vi "SYST_PRES.vi"(0 "VISA IN":refnum<visa-resource-name>, 5 "error in":errorcluster) -> (14 "VISA Out":refnum<visa-resource-name>, 19 "error out":errorcluster)   [LabVIEW 2018, in "PNA-X.lvlib"]
doc: "SYSTem:PRESet. The contents of the analyzer's non-volatile memory are not affected by this \ncommand. \n*SRE - Service Request Enable \nBefore reading a status register, bits must be enabled. This command enables bits in the service request \nregister. The current setting is saved in non-volatile memory. See Status Commands and Reading the \nAnalyzer's Status Registers. \n*SRE? - Service Request Enable Query \nReads the current state of the service request enable register. The register is cleared after reading it. The \nreturn value can be decoded using the table in Status Commands. See also Reading the Analyzer's \n1483\n\nStatus Registers. \n*STB? - Status Byte Query \nReads the value of the instrument status byte. The register is cleared only when the registers feeding it \nare cleared. See Status Commands and Reading the Analyzer's Status Registers. \n*TST? - Result of Self-test Query \nReturns the result of a query of the analyzer hardward status. An 0 indicates no failures found. Any \nother value indicates one or more of the following conditions exist. The value returned is the Weight \n(or sum of the Weights) of the existing conditions. For example: \nIf 4 is returned from *TST?, an Overpower condition exists. \nIf 6 is returned, both Unleveled and Overpower conditions exists. \nBit Weight Description Bit is set to 1 when the following conditions exist: \n0 1 Phase Unlock The source has lost phaselock. This could be caused by a \nreference channel open or a hardware failure. \n1 2 Unleveled The source power is unleveled. This could be a source is set \nfor more power than it can deliver at the tuned frequency. Or \nit could be caused by a hardware failure. \n2 4 Not used \n3 8 EE Write Failed An attempted write to the EEPROM has failed. This is \npossibly caused by a hardware failure. \n4 16 YIG Cal Failed The analyzer was unable to calibrate the YIG. Either the \nphaselock has been lost or there has been a hardware failure. \n5 32 Ramp Cal Failed The analyzer was unable to calibrate the analog ramp \ngenerator due to a possible hardware failure. \n6 64 Not used \n*WAI - Wait \nProhibits the instrument from executing any new commands until all pending overlapped commands \nhave been completed. See Understanding Command Synchronization \n1484\n\nAbout Triggering \nAbort Command \nABORt \n(Write-only) Stops all sweeps - then resume per current trigger settings. This command is the same as \nINITtiate:IMMediate (restart) except if a channel is performing a single sweep, ABORt will stop the \nsweep, but not initiate another sweep. \nLearn about Synchronizing the PNA and Controller \nExamples ABOR \nabort \nQuery Syntax Not applicable \nDefault Not applicable \n1485\n\nCalculate:Correction Commands \nControls error correction functions. \nClick on a blue keyword to view the command details. \nSee Also \nExample Programs \nNew Calibrating the PNA Using SCPI \nSynchronizing the PNA and Controller \nSCPI Command Tree \nCritical Note: CALCulate commands act on the selected measurement. You can select one \nmeasurement for each channel using Calc:Par:Select \nCALCulate<cnum>:CORRection:EDELay:MEDium <char> \n(Read-Write) Sets the media used when calculating the electrical delay. \nParameters \n<cnum> Any existing channel number. If unspecified, value is set to 1. \n<num> Choose from: COAX for coaxial medium, WAVEguide for waveguide \nmedium. \nExamples CALC:CORR:EDEL:MED COAX \ncalc3:corr:edelay:medium waveguide \nQuery Syntax CALCulate<cnum>:CORRection:EDELay:MEDium? \nReturn Type Character \nDefault COAX \n1486\n\nCALCulate<cnum>:CORRection:EDELay:TIME <num> \n(Read-Write) Sets the electrical delay for the selected measurement. \nSee Critical Note \nParameters \n<cnum> Channel number of the measurement. There must be a selected measurement \non that channel. If unspecified, <cnum> is set to 1. \n<num> Electrical delay in seconds. Choose any number between: \n-10.00 and 10.00 \nUse SENS:CORR:RVEL:COAX <num> to set Velocity factor. \nExamples CALC1:CORR:EDEL:TIME 1NS \ncalculate2:correction:time 0.5e-12 \nQuery Syntax CALCulate:CORRection:EDELay:TIME? \nReturn Type Numeric \nDefault 0 seconds \nCALCulate<cnum>:CORRection:EDELay:WGCutoff <num> \n(Read-Write) Sets the waveguide cutoff frequency used when the electrical delay media is set to \nWAVEguide. (See CALCulate:CORRection:EDELay:MEDium <char>.) \nParameters \n<cnum> Any existing channel number. If unspecified, value is set to 1. \n<num> Waveguide cutoff frequency used with the electrical delay calculation. \nExamples CALC:CORR:EDEL:WGC 18.067 GHz \ncalculate3:correction:edelay:wgcutoff 14.047 ghz \nQuery Syntax CALCulate<cnum>:CORRection:EDELay:WGCutoff? \nReturn Type Numeric \nDefault 45 MHz \nCALCulate<cnum>: CORRection:[STATe] <bool> \n1487\n\n(Read-Write) Turns error correction ON or OFF for the selected measurement on the specified \nchannel. \nTo turn error correction ON or OFF for a channel, use SENS:CORR:STATe. \nSee Critical Note \nParameters \n<cnum> Any existing channel number. If unspecified, value is set to 1 \n<bool> Correction state. Choose from: \n0 - Correction OFF \n1 - Correction ON \nExamples CALC:CORR ON \ncalculate:correction:state off \nQuery Syntax CALCulate<cnum>: CORRection: STATe? \nReturn Type Boolean \nDefault Not Applicable \nCALCulate<cnum>:CORRection:TYPE <string> \n(Read-Write) Sets the Cal Type for the selected measurement on the specified channel. This is used \nwhen a Cal Set is applied. Learn more about applying Cal Types. \nUse SENS:CORR:TYPE:CAT? to list the Cal Types in the PNA. \nUse SENS:CORR:CSET:TYPE:CAT? to list the Cal Types contained in the active Cal Set for the channel. \nUse SENS:CORR:COLL:METH to set the Cal type to perform a new calibration, \nSee Critical Note \nParameters \n<cnum> Any existing channel number. If unspecified, value is set to 1 \n<string> (String) Cal type. Case sensitive. Use one of the following: \nFor Full Calibrations: \nThis command does not distinguish between TRL and SOLT. The same \nnumber of error terms is applied for both Cal Types. \n1488\n\n\"Full n Port (x,y,z...)\" \nwhere\nn = the number of ports to calibrate \nx,y,z = the port numbers to calibrate \nFor example: \n\"Full 7 Port(2,3,4,5,6,7,8)\" \nFor Response Calibrations: \n\"Response(param)\" OR \n\"ResponseAndIsolation(param)\" \nWhere param = \nS-parameter. For example\" \n\"Response(S21)\" \n\"ResponseAndIsolation(A/R)\" \nSingle or ratioed receivers using either logical receiver notation or physical \nreceiver notation. For example: \n\"Response(A)\" \n\"ResponseAndIsolation(a3/b4)\" \nFor FCA Calibrations: \n\"Scalar Mixer Cal\" \n\"SMC with NO Output Match Correction\" \n\"SMC with NO Input Match Correction\" \n\"SMC with NO Match Correction\" \n\"Vector Mixer Cal\" \n\"Characterize Mixer Only\" \nYou can also use a ClassID or GUID. For example: \n1489\n\nCLSID - \"VectorMixerCal.VCMCType\" \nGUID - \"{2061767B-0FE2-4F6F-86D0-9AB332B18DA5}\" \nExamples CALC:CORR:TYPE \"Vector Mixer Cal\" \nQuery Syntax CALCulate<cnum>:CORRection:TYPE? \nReturn Type String \nDefault Not Applicable \nCALCulate<cnum>:CORRection:OFFSet[:MAGNitude] <num> Superseded \nNote: This command is replaced with SENS:CORR:RPOWer:OFFSet[:AMPLitude]. \nTo set data trace magnitude offset, use CALC:OFFS:MAGN \nThis command does NOT function for FCA measurements. \nSee an example of a Receiver Power Calibration. \n(Read-Write) \nFor Receiver Power Calibration, specifies the power level to which the selected (unratioed) \nmeasurement data is to be adjusted. This command applies only when the selected measurement is of \nunratioed power. \nParameters \n<cnum> Channel number of the measurement. There must be a selected measurement \non that channel. If unspecified, <cnum> is set to 1. \n<num> Cal power level in dBm. No limits are enforced on this value, but the PNA \nreceivers themselves have maximum and minimum power specifications (that \nmay differ between PNA models) which this value must comply with for a \nvalid receiver power cal. \nExamples CALC:CORR:OFFS 10DBM \ncalculate1:correction:offset:magnitude maximum \nQuery Syntax CALCulate<cnum>:CORRection:OFFSet[:MAGNitude]? \nReturn Type Numeric \nDefault 0dBm \nCALCulate<cnum>:CORRection:OFFSet:PHASe <num>[<char>] Superseded \n1490\n\nNote: This command is replaced with CALC:OFFS:PHASe \n(Read-Write) Sets the phase offset for the selected measurement. \nParameters \n<cnum> Channel number of the measurement. There must be a selected measurement \non that channel. If unspecified, <cnum> is set to 1. \n<num> Offset phase value. Choose any number between: \n-360 and 360 \n<char> \nUnits for phase. OPTIONAL. Choose either: \nDEG - Degrees (default) \nRAD - Radians \nExamples CALC:CORR:OFFS:PHAS 10 \ncalculate:correction:offset:phase 20rad \nQuery Syntax CALCulate:CORRection:OFFSet:PHASe? \nReturn Type Numeric, returned value always in degrees \nDefault 0 degrees \nLast modified: \n9/12/06 MQ Modified Calc:Corr for multiport. \n1491\n\nCalculate:Custom Commands \nProvides capability to create and modify Frequency Converter Application (opt 083) measurements. \nSee Also \nExample Programs \nSynchronizing the PNA and Controller \nSCPI Command Tree \nCALCulate<cnum>:CUSTom:DEFine <Mname>, <type> [,param] \n(Write-only) Creates a custom measurement. The custom measurement is not automatically \ndisplayed. You must also do the following: \nUse DISP:WIND:STATe to create a window if it doesn't already exist.� \nUse DISP:WIND:TRAC:FEED to display the measurement \nSelect the measurement (CALC:PAR:SEL) before making additional settings. \nSee an example using this command to create a VMC and SMC measurement \nParameters \n<cnum> Any existing channel number. If unspecified, value is set to 1. \n<Mname> Name of the measurement. Any non-empty, unique string, enclosed in quotes. \n<type> String. The type of custom measurement. Choose from: \n\"Vector Mixer/Converter\" \n\"Scalar Mixer/Converter\" \nThese arguments are new with PNA release 6.0. The old arguments are still \nsupported. \n[param] String. Optional parameter specifies the measurement parameter to create. \n1492\n\nType Valid Parameters: \nVector Mixer/Converter \"S11\" \n\"VC21\" \n\"S22\" \nScalar Mixer/Converter \"S11\" \n\"SC21\" \n\"SC12\" \n\"S22\" \n\"Ipwr\" \n\"RevIPwr\" \n\"Opwr\" \n\"RevOPwr\" \nExamples CALC2:CUST:DEF 'My VC21', 'Vector Mixer/Converter','S22' \nQuery Syntax Not applicable \nOverlapped? No \nDefault Not applicable \nCALCulate<cnum>:CUSTom:MODify <param> \n1493\n\n(Write-only) Changes the selected custom measurement to a different parameter. \nSee an example using this command for a VMC and SMC measurement \nParameters \n<cnum> Channel of the custom measurement to be changed. First, select the \nmeasurement using CALC:PAR:SEL. \n<param> Parameter to change the custom measurement to. Select a parameter that is \nvalid for the type of measurement. \nType Valid Parameters \nVMC Measurement \"S11\" \n\"VC21\" \n\"S22\" \nSMC Measurement \"S11\" \n\"SC21\" \n\"SC12\" \n\"S22\" \n\"Ipwr\" \n\"RevIPwr\" \n\"Opwr\" \n\"RevOPwr\" \nExamples SYST:PRES \nCALC2:CUST:DEF 'My VC21', 'Vector Mixer/Converter' \nCALC:PAR:SEL 'My VC21' \nCALC2:CUST:MOD 'S22' \nQuery Syntax Not applicable \nOverlapped? No \nDefault Not applicable \n1494\n\n1495\n\nCalculate:Data Commands \nControls writing and reading PNA measurement data. \nClick on a blue keyword to view the command details. \nSee Also \nExample Programs \nData Access Map \nSynchronizing the PNA and Controller \nTo read receiver data, use CALC:RDATA? \nTo read error terms, use SENS:CORR:CSET:DATA \nTo read SnP measurement data, use CALC:DATA:SNP? \nSCPI Command Tree \nCritical Note: CALCulate commands act on the selected measurement. You can select one \nmeasurement for each channel using Calc:Par:Select \n(Write) CALCulate<cnum>:DATA <char>,<data> \n(Read) CALCulate<cnum>:DATA? <char> \nReads or writes Measurement data, Memory data, or Normalization Divisor data from the Data \nAccess Map location. \nFor Measurement data, use FDATA or SDATA \nFor Memory data, use FMEM or SMEM. When querying memory, you must first store a trace into memory \nusing CALC:MATH:MEMorize. \nFor Normalization Divisor (Receiver Power Cal error term) data, use SDIV \n1496\n\nFor write operations, data type depends on FORM:DATA command. \nNote: The Calc:Data SCORR command to read / write error terms is Superseded with \nSENS:CORR:CSET:DATA. SCORR commands do NOT accommodate greater than 12 error terms. \nSee Critical Note \nParameters \n<cnum> Channel number of the measurement. There must be a selected measurement on that \nchannel. If unspecified, <cnum> is set to 1. \n<char> FDATA Formatted measurement data to or from Data Access Map location \nDisplay (access point 2). \nCorrected data is returned when correction is ON. \nUncorrected data is returned when correction is OFF. \nReturns TWO numbers per data point for Polar and Smith Chart format. \nReturns one number per data point for all other formats. \nFormat of the read data is same as the displayed format. \nSDATA Complex measurement data. \nWrites data to Data Access Map location Raw Measurement (access \npoint 0). \nWhen writing corrected data, and correction is ON, it will be corrected \nagain, resulting in meaningless data. \nReads data from Apply Error Terms (access point 1). \nReturns TWO numbers per data point. \nCorrected data is returned when correction is ON. \nUncorrected data is returned when correction is OFF. \nFMEM Formatted memory data to or from Data Access Map location Memory \nresult (access point 4). \nReturns TWO numbers per data point for Polar and Smith Chart format. \nReturns one number per data point for all other formats. \nFormat of the read data is same as the displayed format. \nReturned data reflects the correction level (On|OFF) when the data was \n1497\n\nstored into memory. \nSMEM Complex measurement data to or from Data Access Map location \nMemory (access point 3). \nReturns TWO numbers per data point. \nReturned data reflects the correction level (On|OFF) when the data was \nstored into memory. \nReturned data reflects the correction level (On|OFF) when the data was \nstored into memory. \nSDIV Complex data from Data Access Map location Normalization (5). \nReturns TWO numbers per data point. \nIf normalization interpolation is ON and the number of points changes \nafter the initial normalization, the divisor data will then be interpolated. \nWhen querying the normalization divisor, you must first store a divisor \ntrace using CALC:NORMalize[:IMMediate]. \nThe following Calc:Data SCORR command to read / write error terms is Superseded with \nSENS:CORR:CSET:DATA. These SCORR commands do NOT accommodate greater than 12 error \nterms. \nFor 2-Port \nSOLT and \nTRL \ncalibrations \nSpecify this \n<char> \nto get or put this Error Term... \nSCORR1 Forward Directivity \nSCORR2 Forward Source Match \nSCORR3 Forward Reflection Tracking \nSCORR4 Forward Isolation \nSCORR5 Forward Load Match \nSCORR6 Forward Transmission Tracking \nSCORR7 Reverse Directivity \nSCORR8 Reverse Source Match \nSCORR9 Reverse Reflection Tracking \nSCORR10 Reverse Isolation \nSCORR11 Reverse Load Match \nSCORR12 Reverse Transmission Tracking \n1498\n\nEXAMPLE \nCALC:DATA FDATA,Data(x) \ncalculate2:data sdata,data(r,i) \nSee another example using this command. \nReturn Type: Block data \nDefault - Not Applicable \nCALCulate<cnum>:DATA:CUSTom <name>,<data> \n(Read-Write) Reads or writes data from a custom-named measurement buffer. \nSee Critical Note \nParameters \n<cnum> Channel number of the measurement. There must be a selected measurement \non that channel. If unspecified, <cnum> is set to 1. \n<name> Name of the buffer to be read or written \n<data> Data to be read or written to the custom buffer. Format as one number per data \npoint. \nExamples CALC:DATA:CUST 'VectorResult0',0,1,2,3,4,5 'Write \nCALC:DATA:CUST? 'VectorResult0' 'Read \nQuery Syntax CALCulate:DATA:CUSTom? <name> \nReturn Type Depends on Form:Data \nDefault Not Applicable \nCALCulate<cnum>:DATA:CUSTom:CATalog? \n1499\n\n(Read-only) Reads the list of buffer names (comma separated list of string values) available from the \nselected parameter. Specify the measurement using CALCulate:PARameter:SELect. \nSee Critical Note \nParameters \n<cnum> Channel number of the measurement. There must be a selected measurement \non that channel. If unspecified, <cnum> is set to 1. \nExamples CALC:DATA:CUST:CAT? \ncalculate:data:custom:catalog? \nReturn Type String \nDefault Not Applicable \nCALCulate<cnum>:DATA:SNP? <n> Superseded \nNote: This command has been replaced by CALC:DATA:SNP:PORTs? \n(Read-only) Reads SnP data from the selected measurement. Learn more about SnP data. \nNote: This command returns SNP data without header information, and in columns, not in rows as \n.SnP files. This means that the data returned from this command sends all frequency data, then all Sx1 \nmagnitude data, then all Sx1 phase data, and so forth. \nSee Critical Note \nParameters \n<cnum> Channel number of the measurement. There must be a selected measurement \non that channel. If unspecified, <cnum> is set to 1. \n<n> Amount of data to return. If unspecified, <n> is set to 2. The number you \nspecify must be less than or equal to the number of available ports on the PNA. \nChoose from: \n1 (S1P) returns data for the active measurement. \n2 (S2P) returns data for the 2 port parameters associated with the current \nmeasurement. Default. \n3 (S3P) returns data for the 3 port parameters associated with the current \nmeasurement. \n4 (S4P) returns data for the 4 port parameters associated with the current \n1500\n\nmeasurement. \nSnP data can be output using several data formatting options. See \nMMEM:STORe:TRACe:FORMat:SNP. \nSee also MMEM:STOR <file>.<snp> \nExamples CALC:PAR:DEF �MyMeasurement�, S11 \nCALC:PAR:SEL �MyMeasurement� \nCALC:DATA:SNP? 1 \nReturn Type Depends on FORMat:DATA \nDefault Not Applicable \nCALCulate<cnum>:DATA:SNP:PORTs? <\"x,y,z\".> \nNote: This command replaces CALC:DATA:SNP?. This command is more explicit regarding the \ndata to be returned, and works for PNAs with multiport test sets. \n(Read-only) Reads SNP data from the selected measurement for the specified ports. Learn more \nabout SnP data. \nNote: This command returns SNP data without header information, and in columns, not in rows as \n.SnP files. This means that the data returned from this command sends all frequency data, then all Sx1 \nmagnitude data, then all Sx1 phase data, and so forth. \nSee Critical Note \nParameters \n<cnum> Channel number of the measurement. There must be a selected measurement \non that channel. If unspecified, <cnum> is set to 1. \n<\"x,y,z\"> Comma or space delimited port numbers for which data is requested, enclosed \nin quotes. \nSnP data can be output using several data formatting options. See \nMMEM:STORe:TRACe:FORMat:SNP. \nExamples CALC:DATA:SNP:PORTs? \"1,2,4,5,7\" 'read data for these ports \nReturn Type Depends on FORMat:DATA \nDefault Not Applicable \n1501\n\nCALCulate<cnum>:DATA:SNP:PORTs:SAVE <\"x,y,z\">,<filename> \nNote: This command replaces MMEM:STOR sNp. This command is more explicit regarding the data \nto be saved, and works for PNAs with multiport test sets. \n(Write-only) Saves sNp data from the selected measurement for the specified ports. \nLearn more about SNP data. \nSee Critical Note \nParameters \n<cnum> Channel number of the measurement. There must be a selected measurement \non that channel. If unspecified, <cnum> is set to 1. \n<\"x,y,z\"> String Comma or space delimited port numbers for which data is requested, \nenclosed in quotes. \n<filename> String Path, filename, and suffix of location to store the sNp data. The suffix \nis not checked for accuracy. If saving 2 ports, specify \"filename.s2p\"; If saving \n4 ports, specify \"filename.s4p.\", and so forth. \nSnP data can be output using several data formatting options. See \nMMEM:STORe:TRACe:FORMat:SNP. \nExamples CALC:DATA:SNP:PORTs:Save '1,2,4','C:/Program \nFiles/Agilent/Network Analyzer/Documents/MyData.s3p' \nReturn Type Depends on FORMat:DATA \nDefault Not Applicable \nLast modified: \nApril 26, 2007 Added clarification to Calc:Data SDATA \n9/18/06 MQ Added two SNP Ports commands for multiport \n1502\n\nCalculate:Equation Commands \nControls Equation Editor capabilities. \nClick on a blue keyword to view the command details. \nSee Also \nExample Programs \nLearn about Equation Editor \nSynchronizing the PNA and Controller \nSCPI Command Tree \nCritical Note: CALCulate commands act on the selected measurement. You can select one \nmeasurement for each channel using Calc:Par:Select \nCALCulate<cnum>:EQUation:STATe <bool> \n(Read-Write) Turns ON and OFF the equation on selected measurement for the specified channel. If \nthe equation is not valid, then processing is not performed. Use CALC:EQUation:VALid? to ensure \nthat the equation is valid. \nSee Critical Note \nParameters \n<cnum> Channel number of the measurement. There must be a selected measurement \non that channel. If unspecified, <cnum> is set to 1. \n<bool> ON (or 1) - turns equation ON. \nOFF (or 0) - turns equation OFF. \nExamples CALC:EQU:STAT 1 \ncalculate2:equation:state 0 \nQuery Syntax CALCulate<cnum>:EQUation:STATe? \n1503\n\nReturn Type Boolean \nDefault OFF (0) \nCALCulate<cnum>:EQUation:TEXT <string> \n(Read-Write) Specifies an equation or expression to be used on the selected measurement for the \nspecified channel. \nSee Critical Note \nParameters \n<cnum> Channel number of the measurement. There must be a selected measurement \non that channel. If unspecified, <cnum> is set to 1. \n<string> Any valid equation or expression. See Equation Editor. \nExamples 'Equation (includes '=') \nCALC:EQU:TEXT \"foo=S11/S21\" \n'Expression \ncalculate2:equation:text \"S11/S21\" \nQuery Syntax CALCulate<cnum>:EQUation:TEXT? \nReturn Type String \nDefault Not Applicable \nCALCulate<cnum>:EQUation:VALid? \n1504\n\n(Read-Write) Returns a boolean value to indicate if the current equation on the selected measurement \nfor the specified channel is valid. For equation processing to occur, the equation must be valid and \nON (CALC:EQU:STAT 1). \nSee Critical Note \nParameters \n<cnum> Channel number of the measurement. There must be a selected measurement \non that channel. If unspecified, <cnum> is set to 1. \nExamples CALC:EQU:VAL? \ncalculate2:equation:valid? \nReturn Type Boolean \n1 - equation is valid \n0 - equation is NOT valid \nDefault Not Applicable \n1505\n\nCalculate:Filter Commands \nControls the gating function used in time domain measurements. The gated range is specified with \neither (start / stop) or (center / span) commands. \nClick on a blue keyword to view the command details. \nSee Also \nExample Programs \nLearn about Gating \nSynchronizing the PNA and Controller \nSCPI Command Tree \nCritical Note: CALCulate commands act on the selected measurement. You can select one \nmeasurement for each channel using Calc:Par:Select \nCALCulate<cnum>:FILTer[:GATE]:COUPle:PARameters <num> \n1506\n\nCALCulate<cnum>:FILTer[:GATE]:COUPle:PARameters <num> \n(Read-Write) Specifies the time domain gating parameters to be coupled. The settings for those \nparameters will be copied from the selected measurement to all other measurements on the channel. \nTo enable Trace Coupling, use SENS:COUP:PAR \nTo specify Transform parameters to couple, use CALC:TRAN:COUP:PAR \nLearn more about Time Domain Trace Coupling \nSee Critical Note \nParameters \n<cnum> Channel number of the measurement. There must be a selected measurement \non that channel. If unspecified, <cnum> is set to 1. \n<num> (Numeric) Parameters to couple. To specify more than one parameter, add the \nnumbers. \n1 - Gating Stimulus (Start, Stop, Center, and Span TIME settings.) \n2 - Gating State (ON / OFF) \n4 - Gating Shape (Minimum, Normal, Wide, and Maximum) \n8 - Gating Type (Bandpass and Notch) \nExamples 'To couple all parameters: \nCALC:FILT:COUP:PAR 15 \n'To couple Stimulus and Type: \ncalculate2:filter:gate:couple:parameters 9 \nQuery Syntax CALCulate<cnum>:FILTer:GATE:COUPle:PARameters? \nReturn Type Numeric \nDefault 13 (All parameters except 2 - Gating State) \nCALCulate<cnum>:FILTer[:GATE]:TIME:CENTer <num> \n1507\n\n(Read-Write) Sets the gate filter center time. \nSee Critical Note \nParameters \n<cnum> Channel number of the measurement. There must be a selected measurement \non that channel. If unspecified, <cnum> is set to 1. \n<num> Center time in seconds; Choose any number between: \n� (number of points-1) / frequency span \nNote: This command will accept MIN or MAX instead of a numeric \nparameter. See SCPI Syntax for more information. \nExamples CALC:FILT:GATE:TIME:CENT -5 ns \ncalculate2:filter:time:center maximum \nQuery Syntax CALCulate<cnum>:FILTer[:GATE]:TIME:CENTer? \nReturn Type Numeric \nDefault 0 \nCALCulate<cnum>:FILTer[:GATE]:TIME:SHAPe <char> \n(Read-Write) Sets the gating filter shape when in time domain. \nSee Critical Note \nParameters \n<cnum> Channel number of the measurement. There must be a selected measurement \non that channel. If unspecified, <cnum> is set to 1. \n<char> Choose from \nMAXimum - the widest gate filter available \nWIDE - \nNORMal - \nMINimum - the narrowest gate filter available \nExamples CALC:FILT:GATE:TIME:SHAP MAX \ncalculate2:filter:time:shape normal \nQuery Syntax CALCulate<cnum>:FILTer[:GATE]:TIME:SHAPe? \nReturn Type Character \nDefault NORMal \n1508\n\nCALCulate<cnum>:FILTer[:GATE]:TIME:SPAN <num> \n(Read-Write) Sets the gate filter span time. \nSee Critical Note \nParameters \n<cnum> Channel number of the measurement. There must be a selected measurement \non that channel. If unspecified, <cnum> is set to 1. \n<num> Time span in seconds; Choose any number between: \n0 and 2* [(number of points-1) / frequency span] \nNote: This command will accept MIN or MAX instead of a numeric \nparameter. See SCPI Syntax for more information. \nExamples CALC:FILT:GATE:TIME:SPAN 5 ns \ncalculate2:filter:time:span maximum \nQuery Syntax CALCulate<cnum>:FILTer[:GATE]:TIME:SPAN? \nReturn Type Numeric \nDefault 20 ns \nCALCulate<cnum>:FILTer[:GATE]:TIME:STATe <boolean> \n(Read-Write) Turns gating state ON or OFF. \nSee Critical Note \nNote: Sweep type must be set to LInear Frequency in order to use Transform Gating. \nParameters \n<cnum> Channel number of the measurement. There must be a selected measurement \non that channel. If unspecified, <cnum> is set to 1. \n<boolean> ON (or 1) - turns gating ON. \nOFF (or 0) - turns gating OFF. \nExamples CALC:FILT:TIME:STAT ON \ncalculate2:filter:gate:time:state off \nQuery Syntax CALCulate<cnum>:FILTer[:GATE]:TIME:STATe? \nReturn Type Boolean (1 = ON, 0 = OFF) \nDefault OFF \n1509\n\nCALCulate<cnum>:FILTer[:GATE]:TIME:STARt <num> \n(Read-Write) Sets the gate filter start time. \nSee Critical Note \nParameters \n<cnum> Channel number of the measurement. There must be a selected measurement \non that channel. If unspecified, <cnum> is set to 1. \n<num> Start time in seconds; any number between: \n� (number of points-1) / frequency span \nNote: This command will accept MIN or MAX instead of a numeric \nparameter. See SCPI Syntax for more information. \nExamples CALC:FILT:TIME:STAR 1e-8 \ncalculate2:filter:gate:time:start minimum \nQuery Syntax CALCulate<cnum>:FILTer[:GATE]:TIME:STARt? \nReturn Type Numeric \nDefault 10 ns \nCALCulate<cnum>:FILTer[:GATE]:TIME:STOP <num> \n(Read-Write) Sets the gate filter stop time. \nSee Critical Note \nParameters \n<cnum> Channel number of the measurement. There must be a selected measurement \non that channel. If unspecified, <cnum> is set to 1. \n<num> Stop time in seconds; any number between: \n� (number of points-1) / frequency span \nNote: This command will accept MIN or MAX instead of a numeric \nparameter. See SCPI Syntax for more information. \nExamples CALC:FILT:TIME:STOP -1 ns \ncalculate2:filter:gate:time:stop maximum \nQuery Syntax CALCulate<cnum>:FILTer[:GATE]:TIME:STOP? \nReturn Type Numeric \nDefault 10 ns \n1510\n\nCALCulate<cnum>:FILTer[:GATE]:TIME[:TYPE] <char> \n(Read-Write) Sets the type of gate filter used. \nSee Critical Note \nParameters \n<cnum> Channel number of the measurement. There must be a selected measurement \non that channel. If unspecified, <cnum> is set to 1. \n<char> Choose from: \nBPASs - Includes (passes) the range between the start and stop times. \nNOTCh - Excludes (attenuates) the range between the start and stop times. \nExamples CALC:FILT:TIME BPAS \ncalculate2:filter:gate:time:type notch \nQuery Syntax CALCulate<cnum>:FILTer[:GATE]:TIME[:TYPE]? \nReturn Type Character \nDefault BPAS \n1511\n\nCalculate:Format Command \nCritical Note: CALCulate commands act on the selected measurement. You can select one \nmeasurement for each channel using Calc:Par:Select \nSee Also \nExample using this command. \nLearn About Data Format \nSynchronizing the PNA and Controller \nCALCulate<cnum>:FORMat <char> \n(Read-Write) Sets the display format for the measurement. \nSee Critical Note \nParameters \n<cnum> Channel number of the measurement. There must be a selected measurement \non that channel. If unspecified, <cnum> is set to 1. \n<char> Choose from: \nMLINear \nMLOGarithmic \nPHASe \nUPHase 'Unwrapped phase \nIMAGinary \nREAL \nPOLar \nSMITh \nSADMittance 'Smith Admittance \nSWR \nGDELay 'Group Delay \n1512\n\nExamples CALC:FORM MLIN \ncalculate2:format polar \nQuery Syntax CALCulate<cnum>:FORMat? \nReturn Type Character \nDefault MLINear \n1513\n\nCalculate:FSimulator Commands \nSpecifies settings and fixturing for Balanced Measurements. \nClick a blue keyword to view the command details. \nSee Also \nExample Programs \nSCPI Command Tree \nCALCulate<cnum>:FSIMulator:STATe <bool> \n(Read-Write) Turns all three fixturing functions (de-embedding, port matching, impedance \nconversion) ON or OFF for all ports on the specified channel. Does not affect port extensions. \nNote: This command affects ALL measurements on the specified channel. \nParameters \n<cnum> Channel number of the measurement. There must be a selected measurement \non that channel. If unspecified, <cnum> is set to 1. \n<bool> Choose from: \nON or 1 - Turns Fixturing ON \nOFF or 0 - Turns Fixturing OFF \nExamples CALC:FSIM:STAT 1 \ncalculate2:fsimulator:state 0 \nQuery Syntax CALCulate<cnum>:FSIMulator:STATe? \nReturn Type Boolean \nDefault OFF \n1514\n\n1515\n\nCalculate:Function Commands \nClick on a blue keyword to view the command details. \nSee Also \nExample Programs \nLearn about Trace Statistics \nSynchronizing the PNA and Controller \nSCPI Command Tree \nCritical Note: CALCulate commands act on the selected measurement. You can select one \nmeasurement for each channel using Calc:Par:Select \nCALCulate<cnum>:FUNCtion:DATA? \n(Read-only) Returns the trace statistic data for the selected statistic type for the specified channel. \nSelect the type of statistic with CALC:FUNC:TYPE. \nSee Critical Note \nParameters \n<cnum> Channel number of the measurement. There must be a selected measurement on \nthat channel. If unspecified, <cnum> is set to 1. \nReturn Type Depends on FORM:DATA \nExample CALCulate2:FUNCtion:DATA? \nDefault Not applicable \nCALCulate<cnum>:FUNCtion:DOMain:USER[:RANGe] <range> \n1516\n\n(Read-Write) Sets the range used to calculate trace statistics. Each channel has 16 user ranges. The xaxis \nrange is specified with the CALC:FUNC:DOM:USER:START and STOP commands. \nSee Critical Note \nParameters \n<cnum> Channel number of the measurement. There must be a selected measurement \non that channel. If unspecified, <cnum> is set to 1. \n<range> Range number. Choose from: 0 to 16 \n0 is Full Span of the current x-axis range \n1 to 16 are user-specified ranges \nExamples CALC:FUNC:DOM:USER 4 \ncalculate2:function:domain:user:range 0 \nQuery Syntax CALCulate<cnum>:FUNCtion:DOMain:USER[:RANGe]? \nReturn Type Numeric \nDefault 0 - Full Span \nCALCulate<cnum>:FUNCtion:DOMain:USER:STARt <range>, <start> \n(Read-Write) Sets the start of the specified user-domain range. \nTo apply this range, use CALC:FUNC:DOM:USER \nTo set the stop of the range, use CALC:FUNC:DOM:USER:STOP. \nSee Critical Note \nNote: This command does the same as CALC:MARK:FUNC:DOM:USER:STAR \nParameters \n<cnum> Channel number of the measurement. There must be a selected measurement \non that channel. If unspecified, <cnum> is set to 1. \n<range> Range number that will receive the start value. Choose an integer between 1 \nand 16 \n<start> Start value of the specified range. Choose a real number between: \nthe analyzer's Minimum and Maximum x-axis value. \nExamples CALC:FUNC:DOM:USER:STAR 1,1e9 \ncalculate2:function:domain:user:start 2,2e9 \n1517\n\nQuery Syntax CALCulate<cnum>:FUNCtion:DOMain:USER:STARt? <range> \nReturn Type Numeric \nDefault The analyzer's Minimum x-axis value \nCALCulate<cnum>:FUNCtion:DOMain:USER:STOP <range>, <stop> \n(Read-Write) Sets the stop value of the specified user-domain range. \nTo apply this range, use CALC:FUNC:DOM:USER. \nTo set the start of the range, use CALC:FUNC:DOM:USER:START \nSee Critical Note \nNote: This command does the same as CALC:MARK:FUNC:DOM:USER:STOP \nParameters \n<cnum> Channel number of the measurement. There must be a selected measurement \non that channel. If unspecified, <cnum> is set to 1. \n<range> Range number that will receive the stop value. Choose an integer between 1 \nand 16 \n<stop> Stop value of the specified range. Choose a real number between: \nthe analyzer's Minimum and Maximum x-axis value. \nExamples CALC:FUNC:DOM:USER:STOP 4,5e9 \ncalculate2:function:domain:user:stop 3,8e9 \nQuery Syntax CALCulate<cnum>:FUNCtion:DOMain:USER:STOP? <range> \nReturn Type Numeric \nDefault The analyzer's Maximum x-axis value \nCALCulate<cnum>:FUNCtion:EXECute \n1518\n\n(Write-only) For the active trace of specified channel, executes the statistical analysis specified by the \nCALC:FUNC:TYPE command. \nSee Critical Note \nParameters \n<cnum> Channel number of the measurement. There must be a selected measurement \non that channel. If unspecified, <cnum> is set to 1. \nExamples CALC:FUNC:EXEC \ncalculate2:function:execute \nQuery Syntax Not Applicable \nDefault Not Applicable \nCALCulate<cnum>:FUNCtion:STATistics[:STATe] <ON|OFF> \n(Read-Write) Displays and hides the trace statistics (peak-to-peak, mean, standard deviation) on the \nscreen. \nThe analyzer will display either measurement statistics or Filter Bandwidth statistics; not both. \nSee Critical Note \nParameters \n<cnum> Channel number of the measurement. There must be a selected measurement \non that channel. If unspecified, <cnum> is set to 1. \n<ON|OFF> ON - Displays trace statistics \nOFF - Hides trace statistics \nExamples CALC:FUNC:STAT ON \ncalculate2:function:statistics:state off \nQuery Syntax CALCulate<cnum>:FUNCtion:STATistics[:STATe]? \nReturn Type Boolean (1 = ON, 0 = OFF) \nDefault OFF (0) \nCALCulate<cnum>:FUNCtion:TYPE <char> \n1519\n\n(Read-Write) Sets statistic TYPE that you can then query using CALC:FUNCtion:DATA?. \nNote: In PNA releases 4.2 and prior, this command applied the statistic type to all measurements. \nNow, this command affects only the selected measurement on the specified channel. \nSee Critical Note \nParameters \n<cnum> Channel number of the measurement. There must be a selected measurement \non that channel. If unspecified, <cnum> is set to 1. \n<char> Choose from: \nPTPeak - the difference between the max and min data points on the trace. \nSTDEV - standard deviation of all data points on the trace \nMEAN - mean (average) of all data points on the trace \nMIN - lowest data point on the trace \nMAX - highest data point on the trace \nExamples CALC:FUNC:TYPE PTP \ncalculate2:function:type stdev \nQuery Syntax CALCulate<cnum>:FUNCtion:TYPE? \nReturn Type Character \nDefault PTPeak \n1520\n\nCalc:Limit Commands \nControls the limit segments used for pass / fail testing. \nClick on a blue keyword to view the command details. \nSee Also \nExample Programs \nLearn about Limit Lines \nSynchronizing the PNA and Controller \nSCPI Command Tree \nCritical Note: CALCulate commands act on the selected measurement. You can select one \nmeasurement for each channel using Calc:Par:Select \nCALCulate<cnum>:LIMit:DATA <block> \n(Read-Write) Sets data for limit segments. \nSee Critical Note \nParameters \n<cnum> Channel number of the measurement. There must be a selected measurement \non that channel. If unspecified, <cnum> is set to 1. \n<block> Data for all limit segments in REAL,64 format. The following is the data \nformat for 1 segment: \nType,BegStim, EndStim, BegResp,EndResp \n1521\n\nType Type of limit segment. Choose from \n0 - Off \n1 - Max \n2 - Min \nBegStim Start of X-axis value (freq, power, time) \nEndStim End of X-axis value \nBegResp Y-axis value that corresponds with Start of X-axis value \nEndResp Y-axis value that corresponds with End of X-axis value \nExamples The following writes three max limit segments for a bandpass filter. \n\"CALC:LIM:DATA 1,3e5,4e9,-60,0,1,4e9,7.5e9,0,0,1,7.5e9,9e9,0,- \n30\" \nQuery Syntax CALCulate<cnum>:LIMit:DATA? \nReturn Type Depends on FORM:DATA - All 100 predefined limit segments are returned. \nDefault 100 limit segments - all values set to 0 \nCALCulate<cnum>:LIMit:DISPlay[:STATe] <ON | OFF> \n(Read-Write) Turns the display of limit segments ON or OFF (if the data trace is turned ON). \nSee Critical Note \nParameters \n<cnum> Channel number of the measurement. There must be a selected measurement \non that channel. If unspecified, <cnum> is set to 1. \n<ON | OFF> ON (or 1) - turns the display of limit segments ON. \nOFF (or 0) - turns the display of limit segments OFF. \nExamples CALC:LIM:DISP:STAT ON \ncalculate2:limit:display:state off \nQuery Syntax CALCulate<cnum>:LIMit:DISPlay[:STATe]? \nReturn Type Boolean (1 = ON, 0 = OFF) \nDefault ON \nCALCulate<cnum>:LIMit:SEGMent<snum>AMPLitude:STARt <num> \n1522\n\n(Read-Write) Sets the start (beginning) of the Y-axis amplitude (response) value. \nSee Critical Note \nParameters \n<cnum> Channel number of the measurement. There must be a selected measurement \non that channel. If unspecified, <cnum> is set to 1. \n<snum> Segment number; if unspecified, value is set to 1. \n<num> Choose any number between: -500 and 500 \nDisplay value is limited to the Maximum and Minimum displayed Y-axis \nvalues. \nExamples CALC:LIM:SEGM1:AMPL:STAR 10 \ncalculate2:limit:segment2:amplitude:start 10 \nQuery Syntax CALCulate<cnum>:LIMit:SEGMent<snum>AMPLitude:STARt? \nReturn Type Numeric \nDefault 0 \nCALCulate<cnum>:LIMit:SEGMent<snum>AMPLitude:STOP <num> \n(Read-Write) Sets the stop (end) of the Y-axis amplitude (response) value. \nSee Critical Note \nParameters \n<cnum> Channel number of the measurement. There must be a selected measurement \non that channel. If unspecified, <cnum> is set to 1. \n<snum> Segment number; if unspecified, value is set to 1. \n<num> Choose any number between: -500 and 500 \nDisplay value is limited to the Maximum and Minimum displayed Y-axis \nvalues. \nExamples CALC:LIM:SEGM1:AMPL:STOP 10 \ncalculate2:limit:segment2:amplitude:stop 10 \nQuery Syntax CALCulate<cnum>:LIMit:SEGMent<snum>AMPLitude:STOP? \nReturn Type Numeric \nDefault 0 \n1523\n\nCALCulate<cnum>:LIMit:SEGMent<snum>STIMulus:STARt <num> \n(Read-Write) Sets the start (beginning) of the X-axis stimulus value. \nSee Critical Note \nParameters \n<cnum> Channel number of the measurement. There must be a selected measurement \non that channel. If unspecified, <cnum> is set to 1. \n<snum> Segment number; if unspecified, value is set to 1. \n<num> Choose any number within the X-axis span of the analyzer. \nExamples CALC:LIM:SEGM1:STIM:STAR 10 \ncalculate2:limit:segment2:stimulus:start 10 \nQuery Syntax CALCulate<cnum>:LIMit:SEGMent<snum>STIMulus:STARt? \nReturn Type Numeric \nDefault 0 \nCALCulate<cnum>:LIMit:SEGMent<snum>STIMulus:STOP <num> \n(Read-Write) Sets the stop (end) of the X-axis stimulus value. \nSee Critical Note \nParameters \n<cnum> Channel number of the measurement. There must be a selected measurement \non that channel. If unspecified, <cnum> is set to 1. \n<snum> Segment number; if unspecified, value is set to 1. \n<num> Choose any number within the X-axis span of the analyzer. \nExamples CALC:LIM:SEGM1:AMPL:STOP 10 \ncalculate2:limit:segment2:stimulus:stop 10 \nQuery Syntax CALCulate<cnum>:LIMit:SEGMent<snum>STIMulus:STOP? \nReturn Type Numeric \nDefault 0 \nCALCulate<cnum>:LIMit:SEGMent<snum>:TYPE <char> \n1524\n\n(Read-Write) Sets the type of limit segment. \nSee Critical Note \nParameters \n<cnum> Channel number of the measurement. There must be a selected measurement \non that channel. If unspecified, <cnum> is set to 1. \n<snum> Segment number. Choose any number between: \n1 and 100 \nIf unspecified, value is set to 1. \n<char> Choose from: \nLMAX - a MAX limit segment. Any response data exceeding the MAX value \nwill fail. \nLMIN - a MIN limit segment. Any response data below the MIN value will \nfail. \nOFF - the limit segment (display and testing) is turned OFF. \nExamples CALC:LIM:SEGM:TYPE LMIN \ncalculate2:limit:segment3:type lmax \nQuery Syntax CALCulate<cnum>:LIMit:SEGMent<snum>:TYPE? \nReturn Type Character \nDefault OFF \nCALCulate<cnum>:LIMit:SOUNd[:STATe] <ON | OFF> \n(Read-Write) Turns limit testing fail sound ON or OFF. \nSee Critical Note \nParameters \n<cnum> Channel number of the measurement. There must be a selected measurement \non that channel. If unspecified, <cnum> is set to 1. \n<ON | OFF> ON (or 1) - turns sound ON. \nOFF (or 0) - turns sound OFF. \nExamples CALC:LIM:SOUN ON \ncalculate2:limit:sound:state off \nQuery Syntax CALCulate<cnum>:LIMit:SOUNd[:STATe]? \nReturn Type Boolean (1 = ON, 0 = OFF) \nDefault OFF \n1525\n\nCALCulate<cnum>:LIMit:STATe <ON | OFF> \n(Read-Write) Turns limit segment testing ON or OFF. \nUse CALC:LIM:DISP to turn ON and OFF the display of limit segments. \nIf using Global Pass/Fail status, trigger the PNA AFTER turning Limit testing ON. \nSee Critical Note \nParameters \n<cnum> Channel number of the measurement. There must be a selected measurement \non that channel. If unspecified, <cnum> is set to 1. \n<ON | OFF> ON (or 1) - turns limit testing ON. \nOFF (or 0) - turns limit testing OFF. \nExamples CALC:LIM:STAT ON \ncalculate2:limit:state off \nQuery Syntax CALCulate<cnum>:LIMit:STATe? \nReturn Type Boolean (1 = ON, 0 = OFF) \nDefault OFF \n1526\n\nCalculate:Marker Commands \nControls the marker settings used to remotely output specific data to the computer. \nClick on a blue keyword to view the command details. \nSee Also \nExample Programs \nSee Marker Readout number and size commands. \nLearn about Markers \nSynchronizing the PNA and Controller \nSCPI Command Tree \nCritical Note: CALCulate commands act on the selected measurement. You can select one \nmeasurement for each channel using Calc:Par:Select \nNote: The Reference Marker is Marker Number 10 \nCALCulate<cnum>:MARKer:AOFF \n1527\n\n(Write-only) Turns all markers off for selected measurement. \nSee Critical Note \nParameters \n<cnum> Channel number of the measurement. There must be a selected measurement \non that channel. If unspecified, <cnum> is set to 1. \nExamples CALC:MARK:AOFF \ncalculate2:marker:aoff \nQuery Syntax Not applicable \nDefault Not applicable \nCALCulate<cnum>:MARKer:BWIDth <num> \n(Read-Write) Turns on and sets markers 1 through 4 to calculate filter bandwidth. The <num> \nparameter sets the value below the maximum bandwidth peak that establishes the bandwidth of a \nfilter. For example, if you want to determine the filter bandwidth 3 db below the bandpass peak value, \nset <num> to -3. \nThis feature activates markers 1 through 4. To turn off these markers, either turn them off individually \nor turn them All Off. \nThe analyzer screen will show either Bandwidth statistics OR Trace statistics; not both. \nTo search a User Range with the bandwidth search, first activate marker 1 and set the desired User \nRange. Then send the CALC:MARK:BWID command. The user range used with bandwidth search \nonly applies to marker 1 searching for the max value. The other markers may fall outside the user \nrange. \nSee Critical Note \nParameters \n<cnum> Channel number of the measurement. There must be a selected measurement \non that channel. If unspecified, <cnum> is set to 1. \n<num> Target value below filter peak. Choose any number between :-500 and 500 \nExamples CALC:MARK:BWID -3 \ncalculate2:marker:bwidth -2.513 \nQuery Syntax CALCulate<cnum>:MARKer:BWIDth? \nReturns the results of bandwith search: \n1528\n\nReturn Type Numeric - Four Character values separated by commas: bandwidth, center \nFrequency, Q, loss. \nDefault -3 \nCALCulate<cnum>:MARKer<mkr>:COUPling[:STATe]<ON|OFF> \n(Read-Write) Sets and Reads the state of Coupled Markers (ON and OFF) \nSee Critical Note \nParameters \n<cnum> Channel number of the measurement. There must be a selected measurement \non that channel. If unspecified, <cnum> is set to 1. \n<mkr> Any existing marker number from 1 to 10; if unspecified, value is set to 1. \n<ON|OFF> False (0) - Turns Coupled Markers OFF \nTrue (1) - Turns Coupled Markers ON \nExamples CALC:MARK:COUP ON \ncalculate2:marker8:coupling off \nQuery Syntax CALCulate<cnum>:MARKer<mkr>:COUPling:[STATe]? \nReturn Type Boolean (1 = ON, 0 = OFF) \nDefault OFF \nCALCulate<cnum>:MARKer<mkr>:DELTa <ON|OFF> \n1529\n\n(Read-Write) Specifies whether marker is relative to the Reference marker or absolute. \nNote: The reference marker must already be turned ON with CALC:MARK:REF:STATE. \nSee Critical Note \nParameters \n<cnum> Channel number of the measurement. There must be a selected measurement \non that channel. If unspecified, <cnum> is set to 1. \n<mkr> Any existing marker number from 1 to 10; if unspecified, value is set to 1. \n<ON|OFF> ON (or 1) - Specified marker is a Delta marker \nOFF (or 0) - Specified marker is an ABSOLUTE marker \nExamples CALC:MARK:DELT ON \ncalculate2:marker8:delta off \nQuery Syntax CALCulate<cnum>:MARKer<mkr>:DELTa? \nReturn Type Boolean (1 = ON, 0 = OFF) \nDefault OFF \nCALCulate<cnum>:MARKer<mkr>:DISCrete <ON|OFF> \n(Read-Write) Makes the specified marker display either a calculated value between data points \n(interpolated data) or the actual data points (discrete data). \nSee Critical Note \nParameters \n<cnum> Channel number of the measurement. There must be a selected measurement \non that channel. If unspecified, <cnum> is set to 1. \n<mkr> Any existing marker number from 1 to 10; if unspecified, value is set to 1. \n<ON|OFF> ON (or 1) - Specified marker displays the actual data points \nOFF (or 0) - Specified marker displays calculated data between the actual data \npoints. \nExamples CALC:MARK:DISC ON \ncalculate2:marker8:discrete off \nQuery Syntax CALCulate<cnum>:MARKer<mkr>:DISCrete? \nReturn Type Boolean (1 = ON, 0 = OFF) \nDefault OFF \n1530\n\nCALCulate<cnum>:MARKer<mkr>:DISTance <num> \n(Read-Write) Set or query marker distance on a time domain trace. \nThe Write command moves the marker to the specified distance value. Once moved, you can read the \nY axis value or read the X-axis time value. (Distance is calculated from the X-axis time value.) \nThe Read command reads the distance of the marker. \nIf the marker is set as delta, the WRITE and READ data is relative to the reference marker. \nSee Critical Note \nParameters \n<cnum> Channel number of the measurement. There must be a selected measurement \non that channel. If unspecified, <cnum> is set to 1. \n<mkr> Any existing marker number from 1 to 10; if unspecified, value is set to 1. \n<num> Marker distance in the unit of measure specified with \nCALC:TRAN:TIME:MARK:UNIT \nExamples CALC:MARK:DIST .1 \ncalculate2:marker8:distance 5 \nQuery Syntax CALCulate<cnum>:MARKer<mkr>:DISTance? \nReturn Type Numeric \nDefault Not Applicable \nCALCulate<cnum>:MARKer<mkr>:FORMat <char> \n1531\n\n(Read-Write) Sets the format of the data that will be returned in a marker data query \nCALC:MARK:Y? and the displayed value of the marker readout. The selection does not have to be \nthe same as the measurement's display format. \nSee Critical Note \nParameters \n<cnum> Channel number of the measurement. There must be a selected measurement \non that channel. If unspecified, <cnum> is set to 1. \n<mkr> Any marker number from 1 to 10; if unspecified, value is set to 1 \n<char> Choose from: \nDEFault - The format of the selected measurement \nMLINear - Linear magnitude \nMLOGarithmic - Logarithmic magnitude \nIMPedance - (R+jX) \nADMittance - (G+jB) \nPHASe - Phase \nIMAGinary - Imaginary part (Im) \nREAL - Real part (Re) \nPOLar - (Re, Im) \nGDELay - Group Delay \nLINPhase - Linear Magnitude and Phase \nLOGPhase - Log Magnitude and Phase \nExamples CALC:MARK:FORMat MLIN \ncalculate2:marker8:format Character \nQuery Syntax CALCulate<cnum>:MARKer<mkr>:FORMat? \nReturn Type Character \nDefault DEFault \nCALCulate<cnum>:MARKer<mkr>:FUNCtion:APEak:EXCursion <num> \n1532\n\n(Read-Write) Sets amplitude peak excursion for the specified marker. The Excursion value determines \nwhat is considered a \"peak\". This command applies to marker peak searches (Next peak, Peak Right, \nPeak Left). \nSee Critical Note \nParameters \n<cnum> Channel number of the measurement. There must be a selected measurement \non that channel. If unspecified, <cnum> is set to 1. \n<mkr> Any existing marker number from 1 to 10; if unspecified, value is set to 1. \n<num> Excursion value. Choose any number between -500 and 500. \nNote: This command will accept MIN or MAX instead of a numeric \nparameter. See SCPI Syntax for more information. \nExamples CALC:MARK:FUNC:APE:EXC 10 \ncalculate2:marker8:function:apeak:excursion maximum \nQuery Syntax CALCulate<cnum>:MARKer<mkr>:FUNCtion:APEak:EXCursion? \nReturn Type Numeric \nDefault 3 \nCALCulate<cnum>:MARKer<mkr>:FUNCtion:APEak:THReshold <num> \n(Read-Write) Sets peak threshold for the specified marker. If a peak (using the criteria set with \n:EXCursion) is below this reference value, it will not be considered when searching for peaks. This \ncommand applies to marker peak searches (Next peak, Peak Right, Peak Left). \nSee Critical Note \nParameters \n<cnum> Channel number of the measurement. There must be a selected measurement \non that channel. If unspecified, <cnum> is set to 1. \n<mkr> Any marker number from 1 to 10; if unspecified, value is set to 1 \n<num> Threshold value.Choose any number between -500 and 500. \nNote: This command will accept MIN or MAX instead of a numeric \nparameter. See SCPI Syntax for more information. \nExamples CALC:MARK:FUNC:APE:THR -40 \ncalculate2:marker8:function:apeak:threshold -55 \n1533\n\nQuery Syntax CALCulate<cnum>:MARKer<mkr>:FUNCtion:APEak:THReshold? \nReturn Type Numeric \nDefault -100 \nCALCulate<cnum>:MARKer<mkr>:FUNCtion:DOMain:USER <range> \n(Read-Write) Assigns the specified marker to a range number. The x-axis travel of the marker is \nconstrained to the range's span. The span is specified with the \nCALC:MARK:FUNC:DOM:USER:START and STOP commands, unless range 0 is specified which \nis the full span of the analyzer. \nEach channel has 16 user ranges. (Trace statistics use the same ranges.) More than one marker can use \na domain range. \nSee Critical Note \nParameters \n<cnum> Channel number of the measurement. There must be a selected measurement \non that channel. If unspecified, <cnum> is set to 1. \n<mkr> Any marker number from 1 to 10; if unspecified, value is set to 1 \n<span> User span. Choose any Integer from 0 to 16 \n0 is Full Span of the analyzer \n1 to 16 are available for user-defined x-axis span \nExamples CALC:MARK:FUNC:DOM:USER 1 \ncalculate2:marker8:function:domain:user 1 \nQuery Syntax CALCulate<cnum>:MARKer<mkr>:FUNCtion:DOMain:USER? \nReturns the user span number that the specified marker is assigned to. \nReturn Type Numeric \nDefault 0 - Full Span \nCALCulate<cnum>:MARKer<mkr>:FUNCtion:DOMain:USER:STARt <start> \n1534\n\n(Read-Write) Sets the start of the span that the specified marker's x-axis span will be constrained to. \nUse CALC:MARK:FUNC:DOM:USER<range> to set range number \nUse CALC:MARK:FUNC:DOM:USER:STOP to set the stop value. \nNote: If the marker is assigned to range 0 (full span), the USER:STARt and STOP commands \ngenerate an error. You cannot set the STARt and STOP values for \"Full Span\". \nNote: This command does the same as CALC:FUNC:DOM:USER:STAR \nSee Critical Note \nParameters \n<cnum> Channel number of the measurement. There must be a selected measurement \non that channel. If unspecified, <cnum> is set to 1. \n<mkr> Any marker number from 1 to 10; if unspecified, value is set to 1 \n<start> The analyzer's Minimum x-axis value \nExamples CALC:MARK:FUNC:DOM:USER:START 500E6 \ncalculate2:marker8:function:domain:user:start 1e12 \nQuery Syntax CALCulate<cnum>:MARKer<mkr>:FUNCtion:DOMain:USER:STARt? \nReturn Type Numeric \nDefault The analyzer's Minimum x-axis value \nCALCulate<cnum>:MARKer<mkr>:FUNCtion:DOMain:USER:STOP <stop> \n(Read-Write) Sets the stop of the span that the marker's x-axis travel will be constrained to. \nUse CALC:MARK:FUNC:DOM:USER<range> to set range number \nUse CALC:MARK:FUNC:DOM:USER:STARt to set the stop value. \nNote: If the marker is assigned to range 0 (full span), the USER:STARt and STOP commands \ngenerate an error. You cannot set the STARt and STOP values for \"Full Span\". \nNote: This command does the same as CALC:FUNC:DOM:USER:STOP \nSee Critical Note \nParameters \n1535\n\n<cnum> Channel number of the measurement. There must be a selected measurement on that \nchannel. If unspecified, <cnum> is set to 1. \n<mkr> Any marker number from 1 to 10; if unspecified, value is set to 1. \n<stop> Stop value of x-axis span; Choose any number between the analyzer's MINimum and \nMAXimum x-axis value. \nExamples CALC:MARK:FUNC:DOM:USER:STOP 500e6 \ncalculate2:marker8:function:domain1:user:stop 1e12 \nQuery \nSyntax \nCALCulate<cnum>:MARKer<mkr>:FUNCtion:DOMain:USER:STOP? \nReturn Type Numeric \nDefault The analyzer's MAXimum x-axis value. \nCALCulate<cnum>:MARKer<mkr>:FUNCtion:EXECute [<func>] \n(Write-only) Immediately executes (performs) the specified search function. If no function is \nspecified, executes the selected function. Select the function with CALC:MARK:FUNCtion:SEL. \nSee Critical Note \nParameters \n<cnum> Channel number of the measurement. There must be a selected measurement \non that channel. If unspecified, <cnum> is set to 1. \n<mkr> Any marker number from 1 to 10; if unspecified, value is set to 1. \n<func> Optional argument. The function that is to be performed. Choose from: \nMAXimum - finds the highest value \nMINimum - finds the lowest value \nRPEak - finds the next valid peak to the right \nLPEak - finds the next valid peak to the left \nNPEak - finds the next highest value among the valid peaks \nTARGet - finds the target value to the right, wraps around to the left \nLTARget - finds the next target value to the left of the marker \nRTARget - finds the next target value to the right of the marker \n1536\n\nExamples CALC:MARK:FUNC:EXEC \ncalculate2:marker2:function:execute maximum \nQuery Syntax Not applicable \nDefault Not applicable \nCALCulate<cnum>:MARKer<mkr>:FUNCtion[:SELect] <char> \n(Read-Write) Sets the search function that the specified marker will perform when executed. To \nexecute (or perform) the function, use: \nCALC:MARK:FUNC:EXEC or \nCALC:MARK:FUNC:TRAC ON to automatically execute the search every sweep. \nSee Critical Note \nParameters \n<cnum> Channel number of the measurement. There must be a selected measurement on \nthat channel. If unspecified, <cnum> is set to 1. \n<mkr> Any marker number from 1 to 10; if unspecified, value is set to 1. \n<char> Marker function. Choose from: \nMAXimum - finds the highest value \nMINimum - finds the lowest value \nRPEak - finds the next valid peak to the right \nLPEak - finds the next valid peak to the left \nNPEak - finds the next highest value among the valid peaks \nTARGet - finds the target value to the right, wraps around to the left \nLTARget - finds the next target value to the left of the marker \nRTARget - finds the next target value to the right of the marker \nExamples CALC:MARK:FUNC MAX \ncalculate2:marker8:function:select ltarget \nQuery Syntax CALCulate<cnum>:MARKer<mkr>:FUNCtion[:SELect]? \nReturn Type Character \nDefault MAX \n1537\n\nCALCulate<cnum>:MARKer<mkr>:TARGet <num> \n(Read-Write) Sets the target value for the specified marker when doing Target Searches with \nCALC:MARK:FUNC:SEL <TARGet | RTARget | LTARget> \nSee Critical Note \nParameters \n<cnum> Channel number of the measurement. There must be a selected measurement \non that channel. If unspecified, <cnum> is set to 1. \n<mkr> Any marker number from 1 to 10; if unspecified, value is set to 1. \n<num> Target value to search for; Units are NOT allowed. \nExamples CALC:MARK:TARG 2.5 \ncalculate2:marker8:target -10.3 \nQuery Syntax CALCulate<cnum>:MARKer<mkr>:TARGet? \nReturn Type Numeric \nDefault 0 \nCALCulate<cnum>:MARKer<mkr>:FUNCtion:TRACking <ON | OFF> \n(Read-Write) Sets the tracking capability for the specified marker. The tracking function finds the \nselected search function every sweep. In effect, turning Tracking ON is the same as doing a \nCALC:MARK:FUNC:EXECute command every sweep. \nSee Critical Note \nParameters \n<cnum> Channel number of the measurement. There must be a selected measurement \non that channel. If unspecified, <cnum> is set to 1. \n<mkr> Any marker number from 1 to 10; if unspecified, value is set to 1. \n<ON | OFF> ON (or 1) - The specified marker will \"Track\" (find) the selected function \nevery sweep. \nOFF (or 0) - The specified marker will find the selected function only when \nthe CALC:MARK:FUNC:EXECute command is sent. \nExamples CALC:MARK:FUNC:TRAC ON \ncalculate2:marker8:function:tracking off \nQuery Syntax CALCulate<cnum>:MARKer<mkr>:FUNCtion:TRACking? \n1538\n\nReturn Type Boolean (1 = ON, 0 = OFF) \nDefault OFF \nCALCulate<cnum>:MARKer:REFerence[:STATe] <ON | OFF> \n(Read-Write) Turns the reference marker (marker 10) ON or OFF. When turned OFF, existing Delta \nmarkers revert to absolute markers. \nSee Critical Note \nParameters \n<cnum> Channel number of the measurement. There must be a selected measurement \non that channel. If unspecified, <cnum> is set to 1. \n<ON | OFF> ON (or 1) - turns reference marker ON \nOFF (or 0) - turns reference marker ON \nExamples CALC:MARK:REF ON \ncalculate2:marker:reference:state OFF \nQuery Syntax CALCulate<cnum>:MARKer:REFerence[:STATe]? \nReturn Type Boolean (1 = ON, 0 = OFF) \nDefault OFF \nCALCulate<cnum>:MARKer:REFerence:X <num> \n(Read-Write) Sets and returns the absolute x-axis value of the reference marker (marker 10). \nSee Critical Note \n<cnum> Channel number of the measurement. There must be a selected measurement \non that channel. If unspecified, <cnum> is set to 1. \n<num> X-axis value. Choose any number within the operating domain of the reference \nmarker. \nExamples CALC:MARK:REF:X 1e9 \ncalculate2:marker:reference:x 1e6 \nQuery Syntax CALCulate<cnum>:MARKer:REFerence:X? \nReturn Type Numeric \n1539\n\nDefault If the first Marker, turns ON in the middle of the X-axis span. If not, turns ON \nat the position of the active marker. \nCALCulate<cnum>:MARKer:REFerence:Y? \n(Read-only) Returns the absolute Y-axis value of the reference marker. \nSee Critical Note \nParameters \n<cnum> Channel number of the measurement. There must be a selected measurement \non that channel. If unspecified, <cnum> is set to 1. \nExamples CALC:MARK:REF:Y? \ncalculate2:marker:reference:y? \nReturn Type Character \nDefault Not applicable \nCALCulate<cnum>:MARKer<mkr>:TYPE <char> 
